vi "Log Error_.vi"(8 "error in":errorcluster, 11 "Error log to file":errorcluster) -> (0 "error out":errorcluster)   [LabVIEW 2019]
doc: "Log Errors."
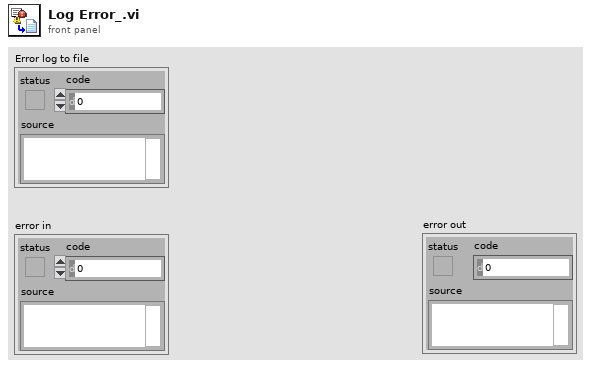
[diagram p1: front panel]
types:
  T1 = enum16{"open", "replace", "create", "open or create", "replace or create", "replace or create with confirmation"}
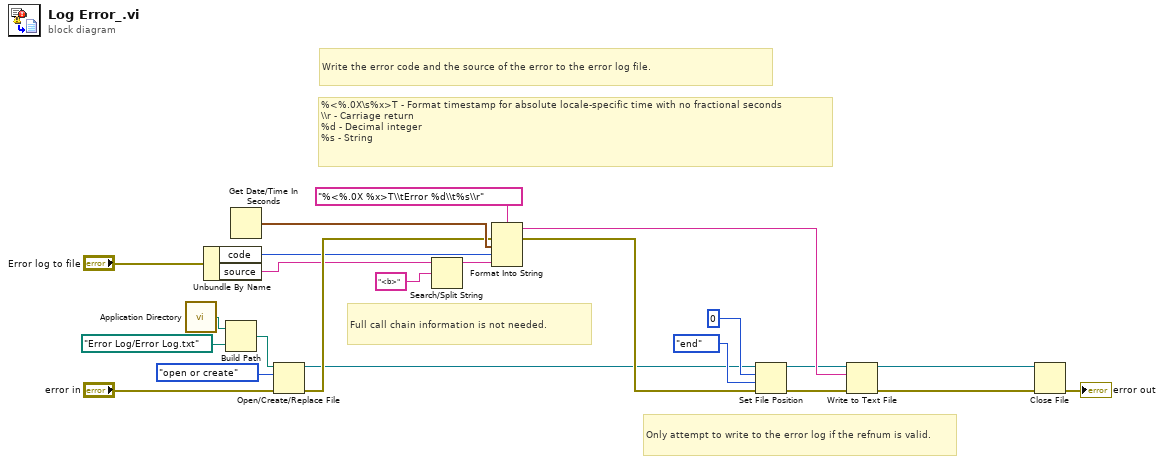
[diagram p0: block diagram]
diagram:
  # "Full call chain information is not needed."
  # "Only attempt to write to the error log if the refnum is valid."
  # "%<%.0X\\s%x>T - Format timestamp for absolute locale-specific time with no fractional seconds\n\\\\r - Carriage return\n%d - Decimal integer\n%s - String"
  # "Write the error code and the source of the error to the error log file."
  n1 = call <vilib>:"Application Directory.vi"() -> ("Application Directory"=w3:path)
  n2 = Unbundle By Name("Error log to file") -> ("code"=w6:i32, "source"=w5:string)
  n3 = Build Path(base path=w3, name or relative path=path "Error Log/Error Log.txt" ("Application Directory")) -> (appended path=w1:path)
  n4 = Get Date/Time In Seconds() -> (seconds since 1Jan1904=w18:timestamp)
  n5 = Open/Create/Replace File(file path (use dialog)=w1, error in="error in", operation (0:open)=T1."open or create") -> (refnum out=w11:refnum<file>, error out=w16:errorcluster)  [unwired: 3 in, 1 out]
  n6 = Search/Split String(string=w5, search string/char (-)="<b>") -> (substring before match=w19:string)  [unwired: 1 in, 2 out]
  n7 = Format Into String(format string="%<%.0X %x>T\\tError %d\\t%s\\r", error in=w16, w18, w6, w19) -> (resulting string=w22:string, error out=w23:errorcluster)  [unwired: 1 in]
  n8 = Set File Position(offset (in bytes) (0)=i64 0, refnum=w11, from (0:start)=enum16{"start", "end", "current"}."end", error in=w23) -> (refnum out=w14:refnum<file>, error out=w15:errorcluster)
  n9 = Write to Text File(file (use dialog)=w14, text=w22, error in=w15) -> (refnum out=w9:refnum<file>, error out=w10:errorcluster)  [unwired: 1 in, 1 out]
  n10 = Close File(refnum=w9, error in=w10) -> (error out=→"error out":errorcluster)  [unwired: 1 out]
